vi "Read UUT_Info.vi"(8 "error in (no error)":errorcluster, 11 "Base Software in":refnum<class "Base Software.lvclass">) -> (0 "error out":errorcluster, 2 "UUT_Info":bool, 3 "Base Software out":refnum<class "Base Software.lvclass">)   [LabVIEW 2019, in "Base Software.lvlib" / "Main.lvlib" / "Base Software.lvclass"]
uses:
  Project/Base Software.lvclass
  Project/Base Software.lvclass/Base Software.ctl
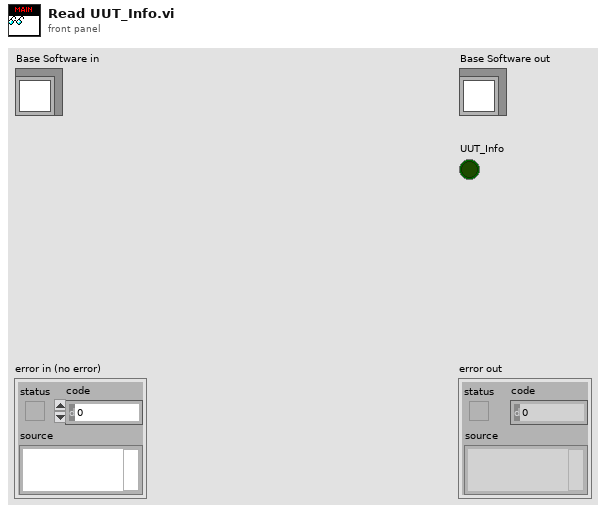
[diagram p1: front panel]
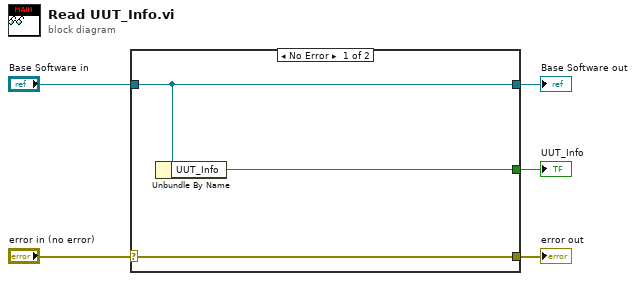
[diagram p0: block diagram]
diagram:
  n1 = case shown="No Error" "error in (no error)" {
    selector: "error in (no error)" -> [w8 w9]
    tunnel: [w8 w9] -> w4
    tunnel: [w7 w10] -> w2
    tunnel: "Base Software in" -> [w7 w10]
    tunnel: [w6 _] -> w1
    frame No Error {
      n2 = Unbundle By Name(w7) -> ("UUT_Info"=w6:bool)
    }
    frame Error {
    }
  }
  "error out" <- w4
  "Base Software out" <- w2
  "UUT_Info" <- w1
